vi "GetColorMatchResultName.vi"(7 "ProjectName":string, 10 "Index":i32, 11 "ROIName":string) -> (3 "ContourResultName":string[](array[string]))   [LabVIEW 2019]
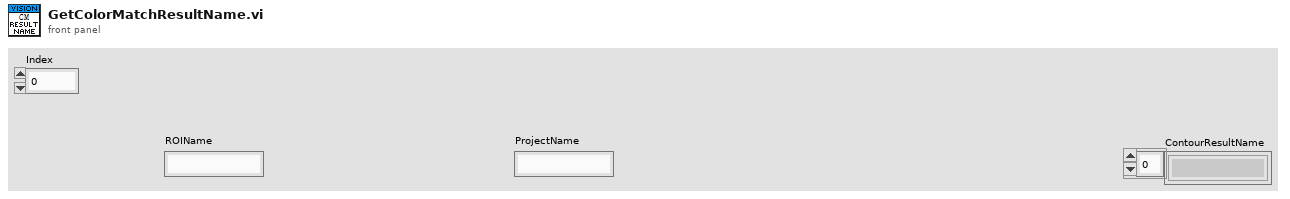
[diagram p1: front panel]
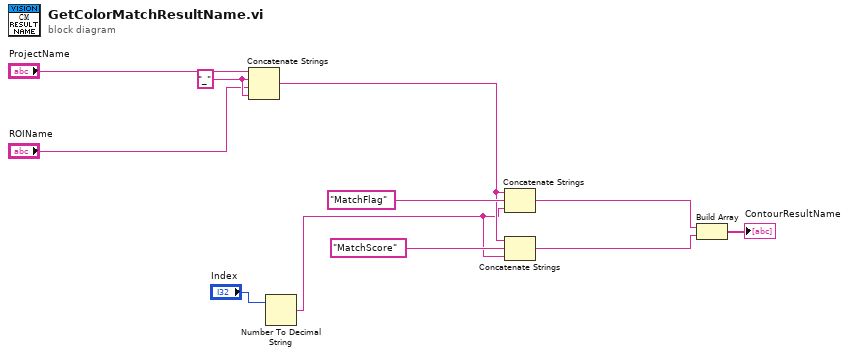
[diagram p0: block diagram]
diagram:
  w11 = "_" ("string")
  n1 = Concatenate Strings("ProjectName", w11, "ROIName", w11) -> (w6:string)
  n2 = Number To Decimal String(number="Index") -> (decimal integer string=w1:string)  [unwired: 1 in]
  n3 = Concatenate Strings(w6, "MatchFlag", w1) -> (w5:string)
  n4 = Concatenate Strings(w6, "MatchScore", w1) -> (w4:string)
  n5 = Build Array(w5, w4) -> (→"ContourResultName":string[])
